vi "proceso5.vi"() -> ()   [LabVIEW 2020]
panel:
  out "proceso 5":T1
  # "pos_inicial_izq = 745\npos_final_izq= 835"
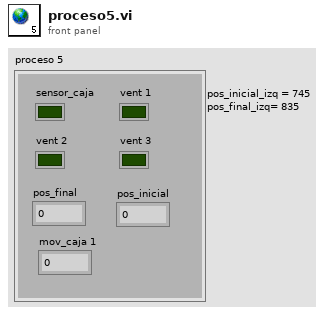
[diagram p1: front panel]
types:
  T1 = cluster{"sensor_caja":bool, "vent 1":bool, "vent 2":bool, "vent 3":bool, "pos_inicial":dbl, "pos_final":dbl, "mov_caja 1":i32}
diagram:
